vi "dvm Open.vi"(8 "error in (no error)":errorcluster, 11 "dvm session in":T1) -> (0 "error out":errorcluster, 2 "idn string":string, 3 "dvm session out":T1)   [LabVIEW 2020]
doc: "Open auxiliary DVM."
uses:
  dvm session.ctl
  dvm type.ctl
  drivers/Fluke 5790A/top_level/F5790 session.ctl
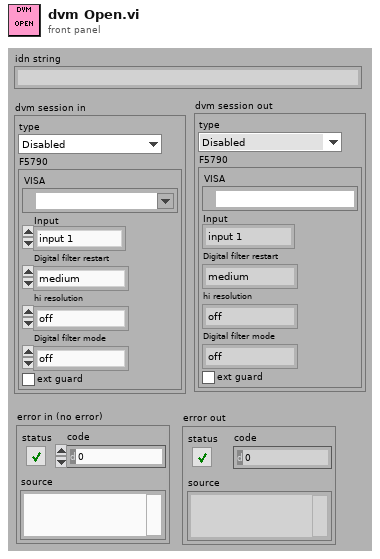
[diagram p1: front panel]
types:
  T1 = typedef "dvm session.ctl" = cluster{"type":T2, "F5790":T3}
  T2 = typedef "dvm type.ctl" = enum16{"Disabled", "Simulated", "Fluke 5790A"}
  T3 = typedef "F5790 session.ctl" = cluster{"VISA":refnum<visa-resource-name>, "Input":enum16{"input 1", "input 2", "wide-band"}, "Digital filter restart":enum16{"medium", "fine", "coarse"}, "hi resolution":enum16{"off", "on"}, "Digital filter mode":enum16{"off", "fast", "medium", "slow"}, "ext guard":bool}
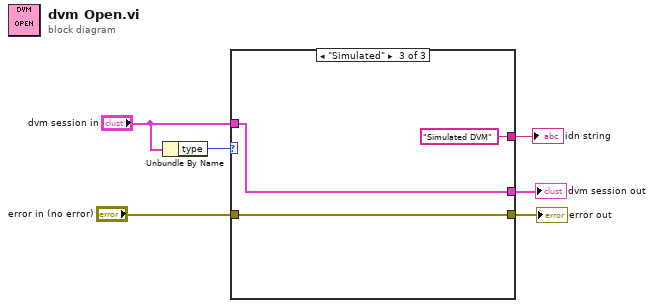
[diagram p0: block diagram]
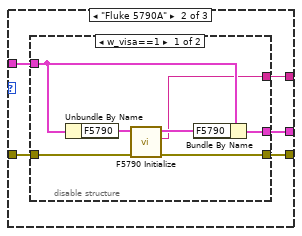
[diagram p3: hidden frame]
diagram:
  n1 = Unbundle By Name("dvm session in") -> ("type"=w6:T2)
  n2 = case shown="\"Simulated\"" w6 {
    tunnel: "dvm session in" -> [w7 w12 w24]
    tunnel: "error in (no error)" -> [w8 w13 w25]
    tunnel: [w8 w11 w25] -> w3
    tunnel: [w7 w10 w24] -> w2
    tunnel: [_ w9 "Simulated DVM" ("ID")] -> w1
    frame "Disabled", Default {
    }
    frame "Fluke 5790A" {
      n3 = disable-structure shown="w_visa==1" {
        disable-tunnel: w13 -> [w20 w22]
        disable-tunnel: w12 -> [w18 w21]
        disable-tunnel: [w16 w22] -> w11
        disable-tunnel: [w15 w21] -> w10
        disable-tunnel: [w14 _] -> w9
        frame condition #0 (active) {
          n4 = Unbundle By Name(w18) -> ("F5790"=w19:T3)
          n5 = call "F5790 Initialize.vi"("error in (no error)"=w20, "F5790 session"=w19) -> ("error out"=w16:errorcluster, "ID"=w14:string, "F5790 session out"=w17:T3)  [unwired: 7 in]
          n6 = Bundle By Name(cluster=w18, "F5790"=w17) -> (w15:T1)
        }
        frame condition #1 {
        }
      }
    }
    frame "Simulated" {
    }
  }
  "error out" <- w3
  "dvm session out" <- w2
  "idn string" <- w1
